vi "3p-abc-dq.vi"(0 "phase value":cluster{"ab":fxp<+/-,24,1>, "bc":fxp<+/-,24,1>}, 1 "estimated theta":fxp<+/-,32,1>) -> (2 "Dout":fxp<+/-,28,4> format="%#.6g", 3 "Qout":fxp<+/-,28,4> format="%#.6g", 4 "sin(theta)":fxp<+/-,32,2> format="%#.5g", 5 "cos(theta)":fxp<+/-,32,2> format="%.31g")   [LabVIEW 2014]
uses:
  <vilib>/Platform/TimedLoop/XDataNode/timing_clust.ctl
  <vilib>/Platform/TimedLoop/XDataNode/nitl_modes.ctl
  <vilib>/Platform/TimedLoop/XDataNode/wakeup.ctl
  <vilib>/rvi/FXPMathLib/FxpSinAndCos/subVIs/nifxpmath_SinAndCos_SimConfig.ctl
  <vilib>/rvi/Emulation/niFpgaSctlEmulationGetInTimedLoop.vi
  <vilib>/rvi/Emulation/niFpgaEmulationReportErrorSimple.vi
  <vilib>/rvi/Emulation/niFpgaGetClockAttributes.vi
  <vilib>/rvi/Emulation/niFpgaCriticalErrorInLSC.vi
  <vilib>/rvi/FXPMathLib/FxpSinAndCos/simVIs/DllFxpSinAndCosTemp_sub.vi
  <vilib>/Platform/TimedLoop/XDataNode/XDataNode.xnode
  <vilib>/rvi/FXPMathLib/FxpSinAndCos/XNode/nifxpmath_SinAndCos.xnode
  <vilib>/rvi/FXPMathLib/FxpMul/XNode/nifxpmath_Multiplier.xnode
  <vilib>/Platform/TimedLoop/XDataNode/XDNodeRunTimeDep.lvlib
  <vilib>/rvi/FXPMathLib/sim/FxpSim.dll
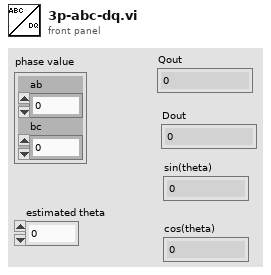
[diagram p1: front panel]
types:
  T1 = typedef "XDNodeRunTimeDep.lvlib/timing_clust.ctl" = cluster{"Expected End [f-1]":u64, "Actual End [f-1]":u64, "Finished Late? [f-1]":bool, "Expected End [i-1]":u64, "Actual End [i-1]":u64, "Finished Late? [i-1]":bool, "Expected Start [i]":u64, "Actual Start [i]":u64, "Expected Start [f]":u64, "Actual Start [f]":u64, "Source Name":string, "Structure Name":string, "Period":i64, "Deadline":i64, "Offset":i64, "Start":i64, "Priority":i32, "Timeout":i32, "Mode":T2, "Wakeup Reason":T3, "Error":errorcluster, "Source Type":string, "Secondary Source Type":string, "Global End Time":u64, "Global Start Time":u64, "Frame Duration":u64, "Iteration Duration":u64, "Assigned CPU":i32, "I/O Scan Engine Mode":u32}
  T2 = typedef "XDNodeRunTimeDep.lvlib/nitl_modes.ctl" = enum32{"No Change", "Process missed periods, maintain original phase", "Discard missed periods, maintain original phase", "Process missed periods, ignore original phase", "Discard missed periods, ignore original phase"}
  T3 = typedef "XDNodeRunTimeDep.lvlib/wakeup.ctl" = enum32{"Normal", "Aborted", "Asynchronous wakeup", "Timing source error", "Timed loop error", "Timeout"}
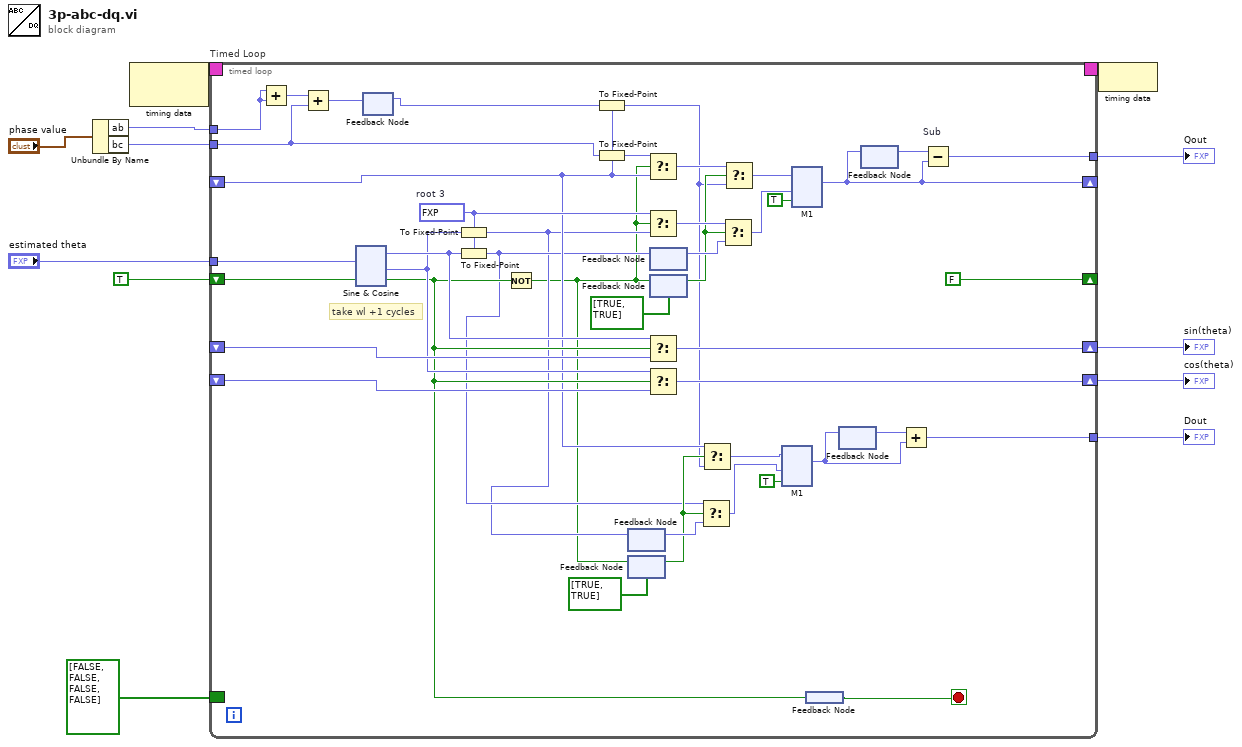
[diagram p0: block diagram]
diagram:
  n1 = Unbundle By Name("phase value") -> ("ab"=w8:fxp<+/-,24,1>, "bc"=w7:fxp<+/-,24,1>)
  n2 = node-c288() -> (w12:T1)  [unwired: 1 in]
  n3 = timed-loop "Timed Loop" {
    timing: w12 -> [_]
    timing-out: [_] -> w11
    tunnel: "estimated theta" -> [w55]
    tunnel: w7 -> [w13]
    shift-right: [w37] -> _
    shift-left: _ -> [w26]
    tunnel: [w48] -> w4
    tunnel: w8 -> [w47]
    shift-right: [w42] -> w3
    shift-left: _ -> [w43]
    shift-right: [w40] -> w2
    shift-left: _ -> [w39]
    shift-right: [FALSE ("input valid")] -> _
    shift-left: TRUE ("input valid") -> [w35]
    border: bool[] [FALSE, FALSE, FALSE, FALSE] -> [_]
    tunnel: [w17] -> w1
    stop <- w32 stop-if-true
    w45 = fxp<+/-,32,2> 1.7320508072152734  # root 3
    # "take wl +1 cycles"
    n4 = Add(x=w47, y=w47) -> (x+y=w16:fxp<+/-,25,2>)
    n5 = Add(x=w16, y=w13) -> (x+y=w15:fxp<+/-,26,3>)
    n6 = xnode "Sine & Cosine"("x (pi)"=w55, "input valid"=w35) -> ("sin(x)"=w44:fxp<+/-,32,2>, "cos(x)"=w41:fxp<+/-,32,2>, "output valid"=w31:bool)  [unwired: 1 in, 1 out]
    n7 = feedback #1() -> (w14:fxp<+/-,26,3>)  [unwired: 1 in]
    n8 = feedback-in #1(w15) -> ()
    n9 = To Fixed-Point(fixed-point type=w45, number=w41) -> (fixed-point=w23:fxp<+/-,32,2>)
    n10 = To Fixed-Point(fixed-point type=w45, number=w44) -> (fixed-point=w24:fxp<+/-,32,2>)
    n11 = Not(x=w31) -> (.not. x?=w22:bool)
    n12 = To Fixed-Point(fixed-point type=w26, number=w14) -> (fixed-point=w25:fxp<+/-,27,3>)
    n13 = To Fixed-Point(fixed-point type=w26, number=w13) -> (fixed-point=w54:fxp<+/-,27,3>)
    n14 = feedback #2() -> (w29:fxp<+/-,32,2>)  [unwired: 1 in]
    n15 = feedback-in #2(w23) -> ()
    n16 = feedback #3(bool[] [TRUE, TRUE]) -> (w27:bool)
    n17 = feedback-in #3(w22) -> ()
    n18 = Select(t=w54, s=w22, f=w26) -> (s? t:f=w53:fxp<+/-,27,3>)
    n19 = Select(t=w45, s=w22, f=w23) -> (s? t:f=w51:fxp<+/-,32,2>)
    n20 = Select(t=w44, s=w31, f=w43) -> (s? t:f=w42:fxp<+/-,32,2>)
    n21 = Select(t=w41, s=w31, f=w39) -> (s? t:f=w40:fxp<+/-,32,2>)
    n22 = feedback-in #4(w24) -> ()
    n23 = feedback #4() -> (w38:fxp<+/-,32,2>)  [unwired: 1 in]
    n24 = feedback #5(bool[] [TRUE, TRUE]) -> (w33:bool)
    n25 = feedback-in #5(w22) -> ()
    n26 = Select(t=w24, s=w27, f=w29) -> (s? t:f=w19:fxp<+/-,32,2>)
    n27 = Select(t=w26, s=w27, f=w25) -> (s? t:f=w21:fxp<+/-,27,3>)
    n28 = Select(t=w51, s=w33, f=w38) -> (s? t:f=w50:fxp<+/-,32,2>)
    n29 = Select(t=w53, s=w33, f=w25) -> (s? t:f=w52:fxp<+/-,27,3>)
    n30 = xnode "M1"("x"=w21, "y"=w19, "input valid"=TRUE) -> ("x*y"=w18:fxp<+/-,27,3>)  [unwired: 1 in, 2 out]
    n31 = xnode "M1"("x"=w52, "y"=w50, "input valid"=TRUE) -> ("x*y"=w37:fxp<+/-,27,3>)  [unwired: 1 in, 2 out]
    n32 = feedback #6() -> (w32:bool)
    n33 = feedback-in #6(w31) -> ()
    n34 = feedback #7() -> (w30:fxp<+/-,27,3>)  [unwired: 1 in]
    n35 = feedback-in #7(w18) -> ()
    n36 = feedback #8() -> (w49:fxp<+/-,27,3>)  [unwired: 1 in]
    n37 = feedback-in #8(w37) -> ()
    n38 = Add(x=w30, y=w18) -> (x+y=w17:fxp<+/-,28,4>)
    n39 = Subtract "Sub"(x=w49, y=w37) -> (x-y=w48:fxp<+/-,28,4>)
  }
  "Qout" <- w4
  "sin(theta)" <- w3
  "cos(theta)" <- w2
  "Dout" <- w1
  n40 = node-c288(w11) -> ()
